vi "Billede_til_String.vi"() -> ()   [LabVIEW 2018]
uses:
  <vilib>/vision/NI_Vision_Development_Module.lvlib
panel:
  in  "File Path":path=path "U:/"
  out "Image Pixels (U8)":u8[][](array[numeric])
  out "Intensity Graph 5":u16[][](graph)
  out "Intensity Graph 3":u8[][](graph)
  out "Original":T1(plugin-control)
  out "Luminance Plane":T1(plugin-control)
  out "Red Plane (as grayscale)":T1(plugin-control)
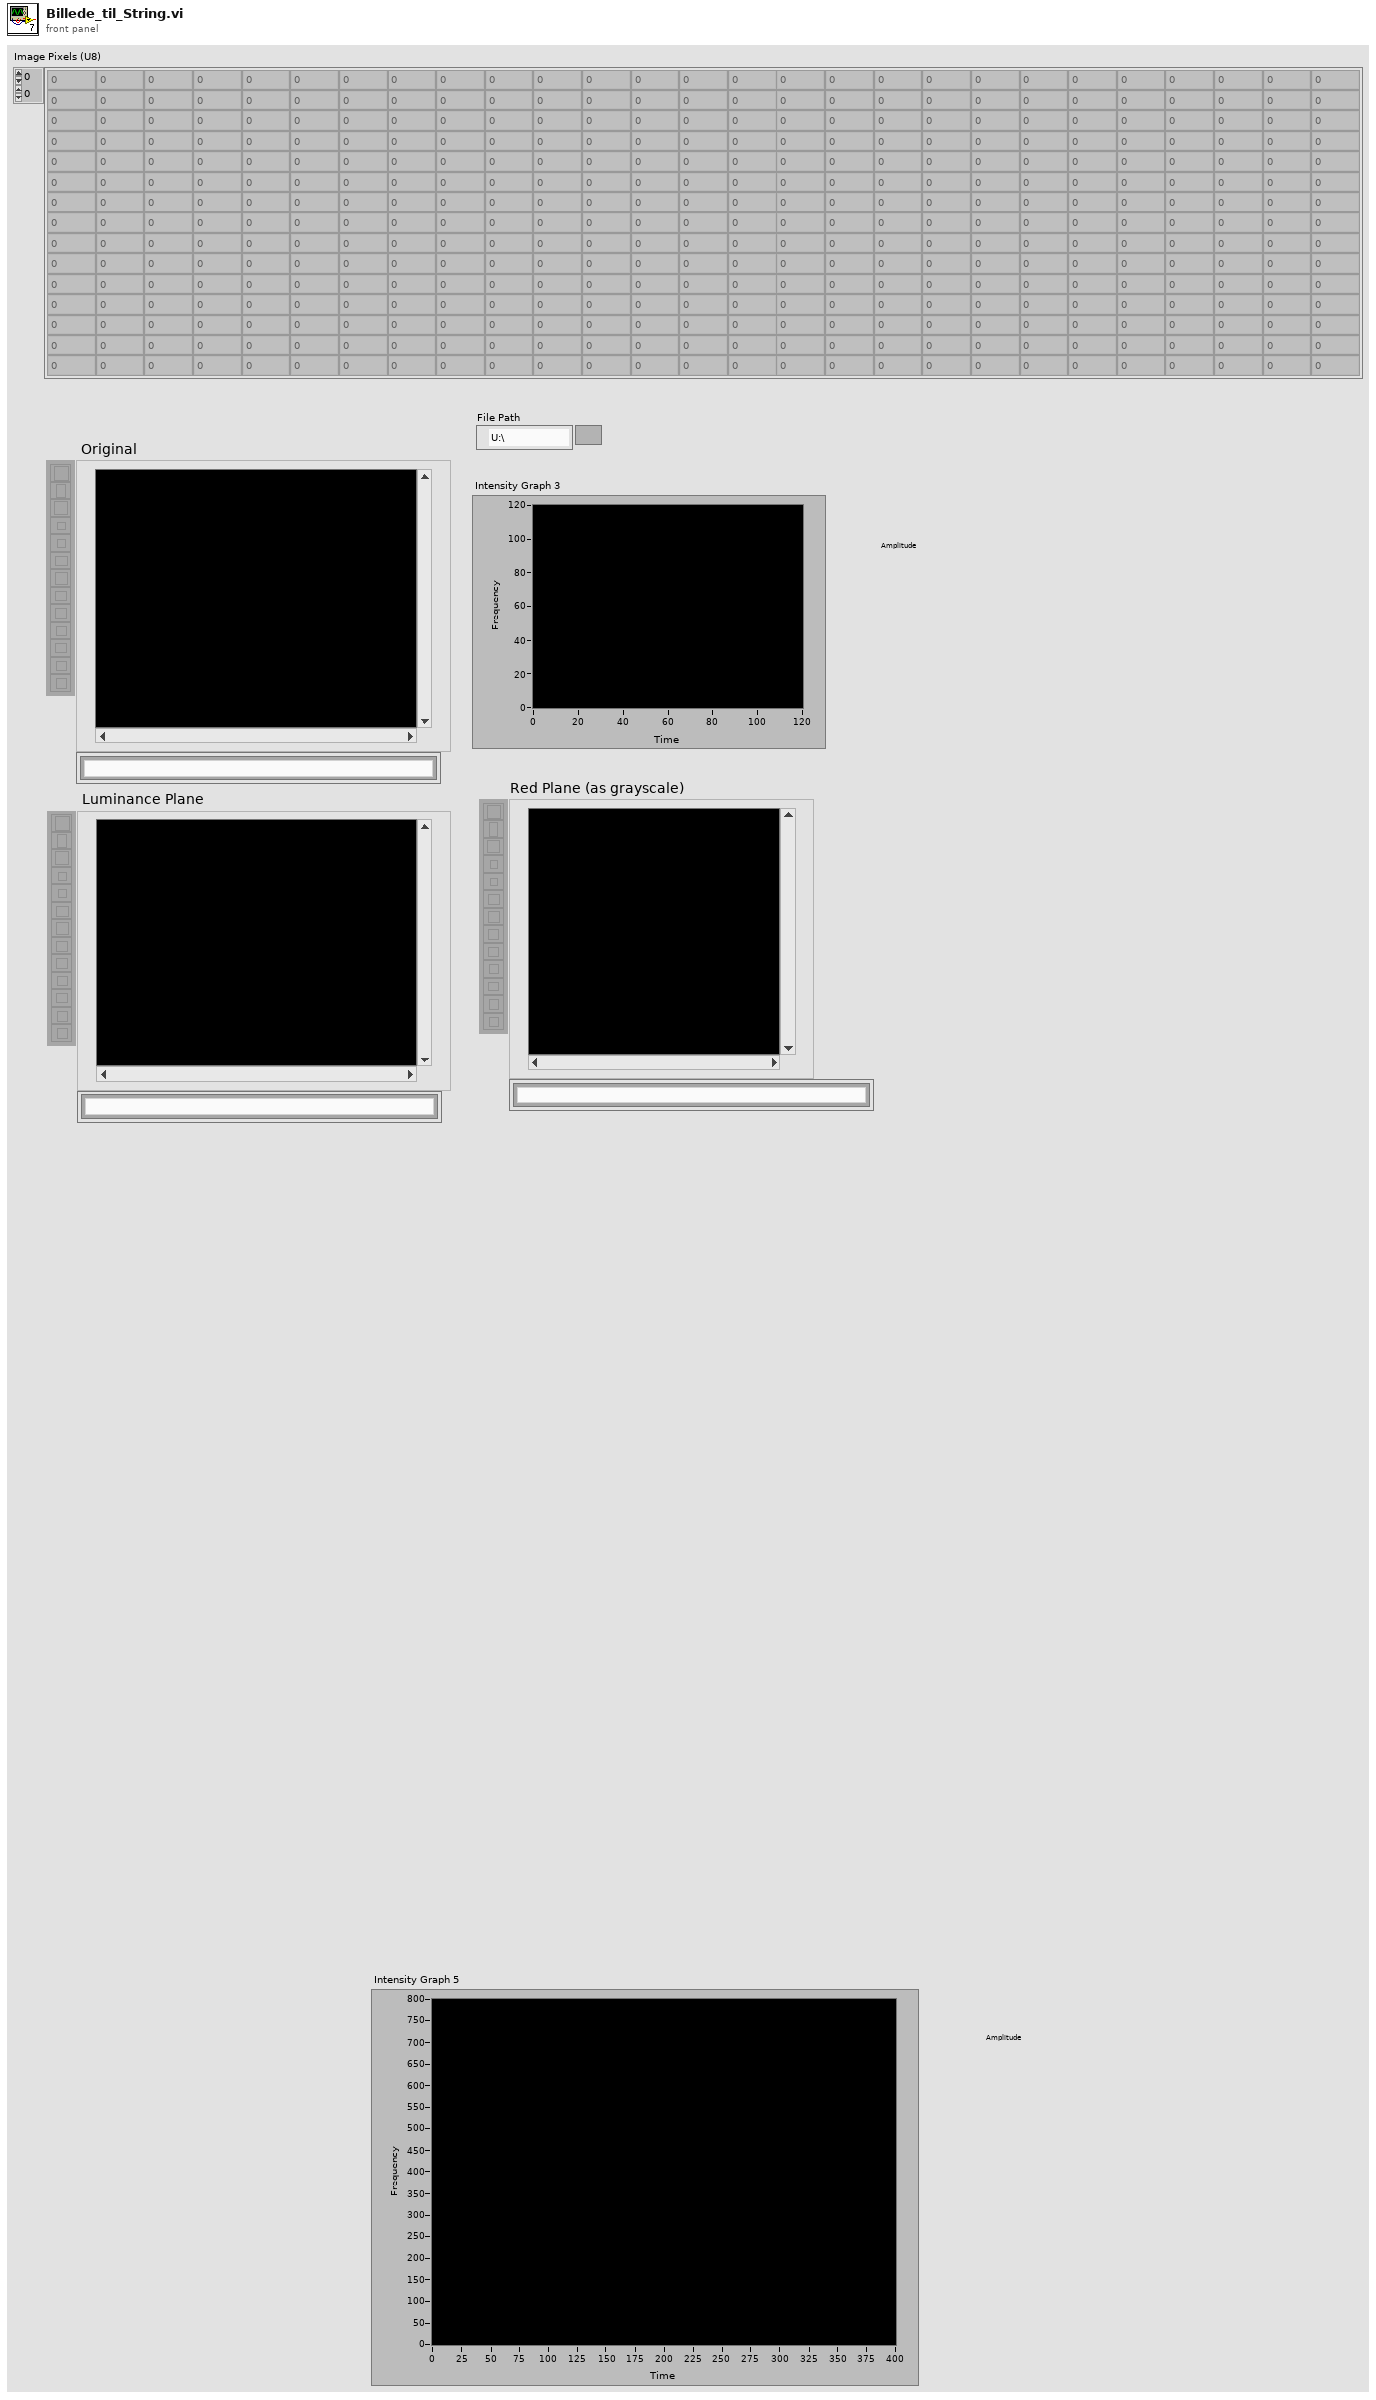
[diagram p1: front panel]
types:
  T1 = typedef "IMAQ Image.ctl" = refnum<image>
  T2 = typedef "Image Type" = u32
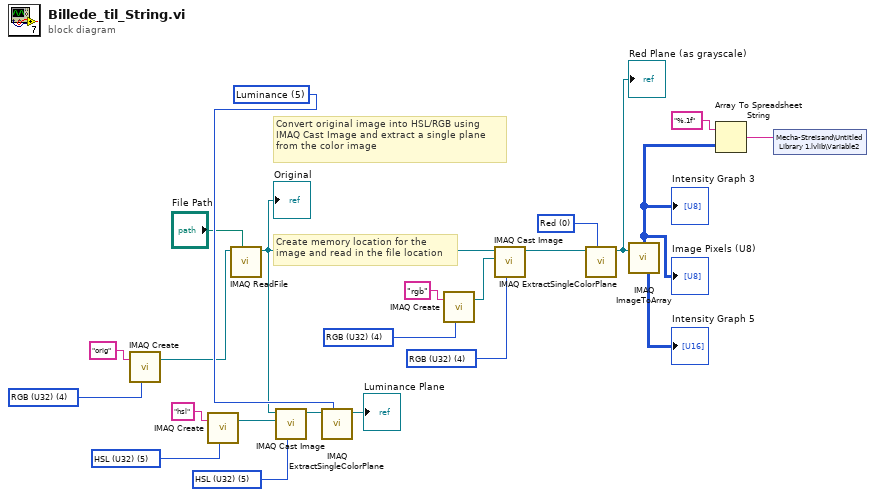
[diagram p0: block diagram]
diagram:
  w7 = T2 4 items=["Grayscale (U8)", "Grayscale (I16)", "Grayscale (SGL)", "Complex (CSG)", "RGB (U32)", "HSL (U32)", "RGB (U64)"] ("Image Type")
  w15 = 0 items=["Red", "Green", "Blue", "Hue", "Saturation", "Luminance", "Value", "Intensity"] ("Color Plane")
  w13 = T2 4 items=["Grayscale (U8)", "Grayscale (I16)", "Grayscale (SGL)", "Complex (CSG)", "RGB (U32)", "HSL (U32)", "RGB (U64)"] ("Image Type")
  w12 = T2 4 items=["Grayscale (U8)", "Grayscale (I16)", "Grayscale (SGL)", "Complex (CSG)", "RGB (U32)", "HSL (U32)", "RGB (U64)"] ("Image Type")
  w17 = 5 items=["Red", "Green", "Blue", "Hue", "Saturation", "Luminance", "Value", "Intensity"] ("Color Plane")
  w19 = T2 5 items=["Grayscale (U8)", "Grayscale (I16)", "Grayscale (SGL)", "Complex (CSG)", "RGB (U32)", "HSL (U32)", "RGB (U64)"] ("Image Type")
  w20 = T2 5 items=["Grayscale (U8)", "Grayscale (I16)", "Grayscale (SGL)", "Complex (CSG)", "RGB (U32)", "HSL (U32)", "RGB (U64)"] ("Image Type")
  # "Convert original image into HSL/RGB using\nIMAQ Cast Image and extract a single plane\nfrom the color image"
  # "Create memory location for the \nimage and read in the file location"
  n1 = call "IMAQ Create"("Image Name"="orig", "Image Type"=w7) -> ("New Image"=w9:T1)  [unwired: 2 in, 2 out]
  n2 = call "IMAQ Create"("Image Name"="hsl", "Image Type"=w20) -> ("New Image"=w22:T1)  [unwired: 2 in, 2 out]
  n3 = call "IMAQ ReadFile"("File Path"="File Path", "Image"=w9) -> ("Image Out"=w6:T1)  [unwired: 3 in, 6 out]
  "Original" <- w6
  n4 = call "IMAQ Cast Image"("Image Type"=w19, "Image Dst"=w22, "Image Src"=w6) -> ("Image Dst Out"=w18:T1)  [unwired: 3 in, 5 out]
  n5 = call "IMAQ ExtractSingleColorPlane"("Color Plane"=w17, "Image Src"=w18) -> ("Image Dst Out"=→"Luminance Plane":T1)  [unwired: 2 in, 7 out]
  n6 = call "IMAQ Create"("Image Name"="rgb", "Image Type"=w12) -> ("New Image"=w10:T1)  [unwired: 2 in, 2 out]
  n7 = call "IMAQ Cast Image"("Image Type"=w13, "Image Dst"=w10, "Image Src"=w6) -> ("Image Dst Out"=w14:T1)  [unwired: 3 in, 5 out]
  n8 = call "IMAQ ExtractSingleColorPlane"("Color Plane"=w15, "Image Src"=w14) -> ("Image Dst Out"=w5:T1)  [unwired: 2 in, 7 out]
  "Red Plane (as grayscale)" <- w5
  n9 = call "IMAQ ImageToArray"("Image"=w5) -> ("Image Pixels (U16)"=→"Intensity Graph 5":u16[][], "Image Pixels (U8)"=w4:u8[][])  [unwired: 3 in, 3 out]
  "Intensity Graph 3" <- w4
  "Image Pixels (U8)" <- w4
  n10 = Array To Spreadsheet String(array=w4, 3:"%.1f" ("format string")) -> (spreadsheet string=w1:string)  [unwired: 1 in]
  n11 = shared-variable "Mecha-Streisand\\Untitled Library 1.lvlib\\Variable2"(w1) -> ()  [unwired: 1 in, 1 out]
